vi "Signal Breakout.vi"(0 "Pumps Enabled":bool[](array[boolean]), 5 "Tank Data":dbl[](array[numeric]), 7 "Intitial Times":dbl[](array[numeric])) -> (4 "Pump Data":T2={"Voltages"=[0.015201568603515625, 0.00335693359375, 0.003021240234375, 0.12260055541992188, 0.06085968017578125, 0.052234649658203125], "PumpCurrent"=[0.015201568603515625, 0.00335693359375, 0.003021240234375, 0.12260055541992188, 0.06085968017578125, 0.052234649658203125], "Speed"=[0.0, 0.0, 0.0, 0.0, 0.0, 0.0], "ControllerCurrent"=[0.015201568603515625, 0.00335693359375, 0.003021240234375, 0.12260055541992188, 0.06085968017578125, 0.052234649658203125], "Pressure"=[0.015201568603515625, 0.00335693359375, 0.003021240234375, 0.12260055541992188, 0.06085968017578125, 0.052234649658203125], "Flow"=[0.0, 0.0, 0.0, 0.125, 0.0625, 0.0625], "Elapsed Time:"=[7.1, 7.1, 7.1, 458133.45, 458138.85000000003, 458126.75]} {"Elapsed Time:" format="%<%H:%M:%S>t"; "Speed" format="%#_4f"; "ControllerCurrent" format="%#.1g"; "Pressure" format="%#.0f"; "Flow" format="%#.0f"; "PumpCurrent" format="%#.1g"; "Voltages" format="%#.0f"}, 6 "Tank Data":T1 {"PS Actual (V):" format="%.2f"; "Temp1" format="%#_2g"; "Temp2" format="%#_2g"}, 8 "Elapsed Time:":dbl[](array[numeric])=[7.1, 7.1, 7.1, 458133.45, 458138.85000000003, 458126.75] format="%<%H:%M:%S>t")   [LabVIEW 2019]
uses:
  Controls/Pump Data.ctl
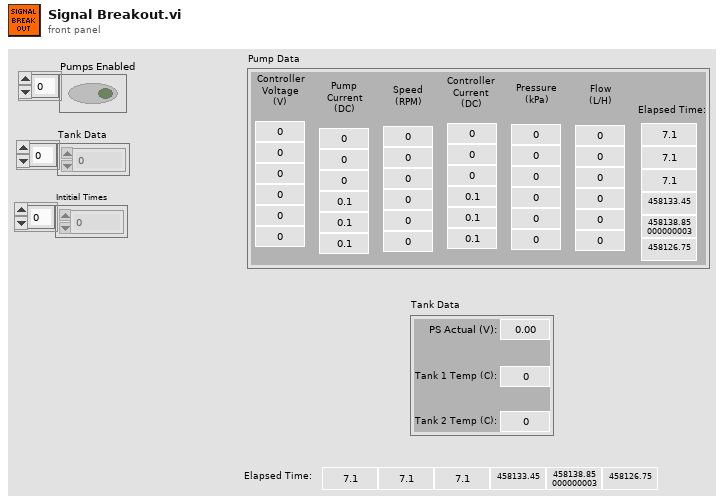
[diagram p1: front panel]
types:
  T1 = cluster{"PS Actual (V):":dbl, "Temp1":dbl, "Temp2":dbl}
  T2 = typedef "Pump Data.ctl" = cluster{"Voltages":dbl[], "PumpCurrent":dbl[], "Speed":dbl[], "ControllerCurrent":dbl[], "Pressure":dbl[], "Flow":dbl[], "Elapsed Time:":dbl[]}
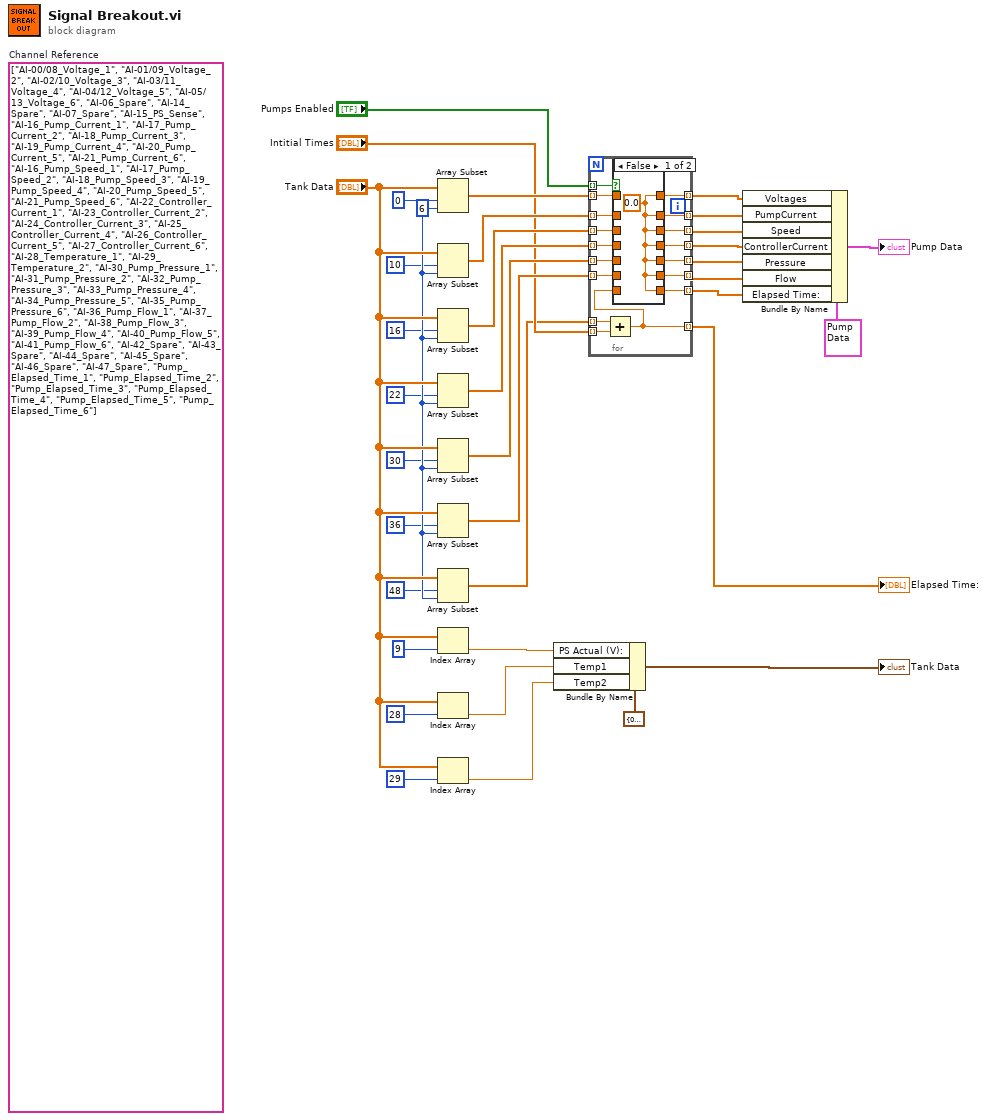
[diagram p0: block diagram]
diagram:
  w34 = 6 ("length")
  (unwired) string[] ["AI-00/08_Voltage_1", "AI-01/09_Voltage_2", "AI-02/10_Voltage_3", "AI-03/11_Voltage_4", "AI-04/12_Voltage_5", "AI-05/13_Voltage_6", "AI-06_Spare", "AI-14_Spare", "AI-07_Spare", "AI-15_PS_Sense", "AI-16_Pump_Current_1", "AI-17_Pump_Current_2", "AI-18_Pump_Current_3", "AI-19_Pump_Current_4", "AI-20_Pump_Current_5", "AI-21_Pump_Current_6", "AI-16_Pump_Speed_1", "AI-17_Pump_Speed_2", "AI-18_Pump_Speed_3", "AI-19_Pump_Speed_4", "AI-20_Pump_Speed_5", "AI-21_Pump_Speed_6", "AI-22_Controller_Current_1", "AI-23_Controller_Current_2", "AI-24_Controller_Current_3", "AI-25_Controller_Current_4", "AI-26_Controller_Current_5", "AI-27_Controller_Current_6", "AI-28_Temperature_1", "AI-29_Temperature_2", "AI-30_Pump_Pressure_1", "AI-31_Pump_Pressure_2", "AI-32_Pump_Pressure_3", "AI-33_Pump_Pressure_4", "AI-34_Pump_Pressure_5", "AI-35_Pump_Pressure_6", "AI-36_Pump_Flow_1", "AI-37_Pump_Flow_2", "AI-38_Pump_Flow_3", "AI-39_Pump_Flow_4", "AI-40_Pump_Flow_5", "AI-41_Pump_Flow_6", "AI-42_Spare", "AI-43_Spare", "AI-44_Spare", "AI-45_Spare", "AI-46_Spare", "AI-47_Spare", "Pump_Elapsed_Time_1", "Pump_Elapsed_Time_2", "Pump_Elapsed_Time_3", "Pump_Elapsed_Time_4", "Pump_Elapsed_Time_5", "Pump_Elapsed_Time_6"]  # Channel Reference
  n1 = Array Subset(array="Tank Data", index=0, length=w34) -> (w24:dbl[])
  n2 = Array Subset(array="Tank Data", index=10, length=w34) -> (w23:dbl[])
  n3 = Array Subset(array="Tank Data", index=16, length=w34) -> (w22:dbl[])
  n4 = Array Subset(array="Tank Data", index=22, length=w34) -> (w21:dbl[])
  n5 = Array Subset(array="Tank Data", index=30, length=w34) -> (w20:dbl[])
  n6 = Array Subset(array="Tank Data", index=36, length=w34) -> (w19:dbl[])
  n7 = Array Subset(array="Tank Data", index=48, length=w34) -> (w8:dbl[])
  n8 = Index Array(array="Tank Data", index=9) -> (element=w6:dbl)
  n9 = Index Array(array="Tank Data", index=28) -> (element=w5:dbl)
  n10 = Index Array(array="Tank Data", index=29) -> (element=w4:dbl)
  n11 = Bundle By Name(cluster=T1 {"PS Actual (V):"=0.0, "Temp1"=0.0, "Temp2"=0.0} ("Tank Data"), "PS Actual (V):"=w6, "Temp1"=w5, "Temp2"=w4) -> (→"Tank Data":T1)
  n12 = for {
    tunnel: w24 -> [w53] mode=indexing
    tunnel: [w52] -> w15 mode=indexing
    tunnel: w23 -> [w51] mode=indexing
    tunnel: w22 -> [w50] mode=indexing
    tunnel: w21 -> [w49] mode=indexing
    tunnel: w20 -> [w48] mode=indexing
    tunnel: w19 -> [w47] mode=indexing
    tunnel: w8 -> [w40] mode=indexing
    tunnel: [w46] -> w14 mode=indexing
    tunnel: [w45] -> w13 mode=indexing
    tunnel: [w44] -> w12 mode=indexing
    tunnel: [w43] -> w11 mode=indexing
    tunnel: [w42] -> w10 mode=indexing
    tunnel: "Pumps Enabled" -> [w41] mode=indexing
    tunnel: "Intitial Times" -> [w39] mode=indexing
    tunnel: [w37] -> w9 mode=indexing
    tunnel: [w38] -> w1 mode=indexing
    n13 = Add(x=w40, y=w39) -> (x+y=w38:dbl)
    n14 = case shown="False" w41 {
      tunnel: w53 -> [_ w61]
      tunnel: [w54 w61] -> w52
      tunnel: w51 -> [_ w60]
      tunnel: w50 -> [_ w59]
      tunnel: w49 -> [_ w58]
      tunnel: w48 -> [_ w57]
      tunnel: w47 -> [_ w56]
      tunnel: [w54 w60] -> w46
      tunnel: [w54 w59] -> w45
      tunnel: [w54 w58] -> w44
      tunnel: [w54 w57] -> w43
      tunnel: [w54 w56] -> w42
      tunnel: [w54 w55] -> w37
      tunnel: w38 -> [_ w55]
      frame False {
        w54 = 0.0
      }
      frame True {
      }
    }
  }
  "Elapsed Time:" <- w1
  n15 = Bundle By Name(cluster=T2 {"Voltages"=[0.0, 0.05908203125, 0.06982421875, 0.05908203125, 0.06982421875, 0.0859375], "PumpCurrent"=[0.0015967955457961394, 0.0015950073791676203, 0.0015981739242389562, 0.0015920643549248493, 0.001590499709124895, 0.0015808510600251774], "Speed"=[0.0, 0.0, 0.0, 0.0, 0.0, 0.0], "ControllerCurrent"=[-20.688123176070036, -20.81007435196841, -20.6654170362211, -20.809705989642936, -20.754042150663764, -20.945938358319978], "Pressure"=[172.64492233694307, 172.85003218327398, 196.83234134789615, 194.272392502873, 196.0868331665868, 197.0256255267641], "Flow"=[114.82946701905468, 115.15906524483574, 115.40397142867363, 115.72441088850422, 113.53169391236554, 111.97984467984668], "Elapsed Time:"=[4074.9003000000002, 4074.9003000000002, 4074.9003000000002, 4074.9003000000002, 4074.9003000000002, 4074.9003000000002]} ("Pump Data"), "Voltages"=w15, "PumpCurrent"=w14, "Speed"=w13, "ControllerCurrent"=w12, "Pressure"=w11, "Flow"=w10, "Elapsed Time:"=w9) -> (→"Pump Data":T2)
